vi "Validate File.vi"(0 "LabVIEW version":string, 7 "Project path":path, 11 "error in (no error)":errorcluster) -> (4 "Warning":string, 15 "error out":errorcluster)   [LabVIEW 2021, in "Converter.lvlib"]
uses:
  Converter.lvlib
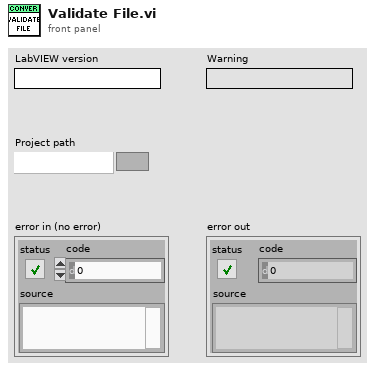
[diagram p1: front panel]
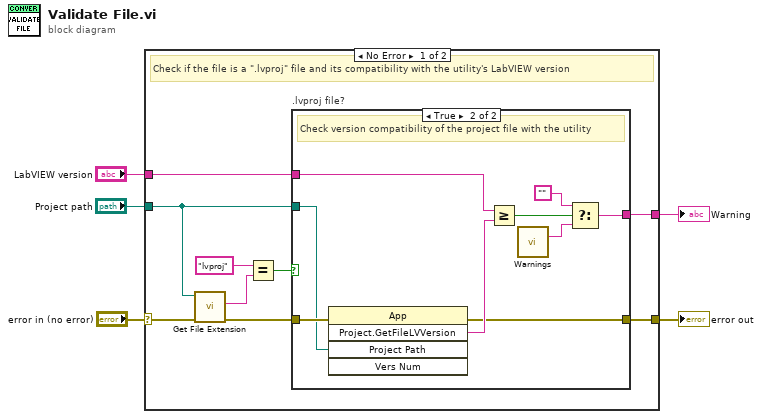
[diagram p0: block diagram]
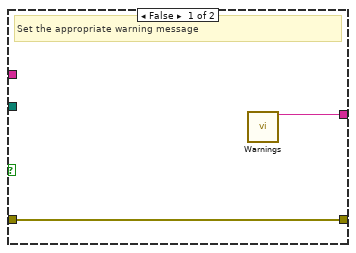
[diagram p2: hidden frame]
diagram:
  n1 = case shown="No Error" "error in (no error)" {
    selector: "error in (no error)" -> [w14 w26]
    tunnel: "Project path" -> [w9 _]
    tunnel: [w7 w26] -> w3
    tunnel: "LabVIEW version" -> [w8 _]
    tunnel: [w6 _] -> w1
    frame No Error {
      # "Check if the file is a \".lvproj\" file and its compatibility with the utility's LabVIEW version"
      n2 = call <vilib>:"Get File Extension.vi"("error in (no error)"=w14, "file"=w9) -> ("error out"=w11:errorcluster, "lowercase file extension"=w13:string)  [unwired: 5 in, 3 out]
      n3 = Equal?(x="lvproj", y=w13) -> (x = y?=w10:bool)
      n4 = case ".lvproj file?" shown="True" w10 {
        tunnel: w11 -> [w15 w25]
        tunnel: w9 -> [_ w17]
        tunnel: w8 -> [_ w24]
        tunnel: [w15 w20] -> w7
        tunnel: [w16 w18] -> w6
        frame False {
          # "Set the appropriate warning message"
          n5 = call "Warnings.vi"() -> ("Invalid project path"=w16:string)  [unwired: 8 in, 7 out]
        }
        frame True {
          # "Check version compatibility of the project file with the utility"
          n6 = invoke class="App" method="Project.GetFileLVVersion"(error in=w25, "Project Path"=w17) -> (error out=w20:errorcluster, "Project.GetFileLVVersion"=w23:string)  [unwired: 3 in, 3 out]
          n7 = Greater Or Equal?(x=w24, y=w23) -> (x >= y?=w22:bool)
          n8 = call "Warnings.vi"() -> ("Incompatible project version"=w21:string)  [unwired: 8 in, 7 out]
          n9 = Select(t="", s=w22, f=w21) -> (s? t:f=w18:string)
        }
      }
    }
    frame Error {
    }
  }
  "error out" <- w3
  "Warning" <- w1
